vi "Convolute (Custom).vi"(6 "Kernel":dbl[][](array[numeric])=[[1.0, 2.0, 1.0], [2.0, 4.0, 2.0], [2.0, 1.0, 2.0]], 7 "Divisor":i32=1, 8 "Image Size in":T1={"Rows (X)"=256, "Colums (Y)"=256}, 9 "Paralellism":i32=2, 10 "Destination Image in":T2=refnum, 11 "Source Image Pixels (U8)":u8[][](array[numeric])) -> (2 "Destination Image Out":T2, 3 "Resulting Image Pixels (U8)":u8[][](array[numeric]))   [LabVIEW 2017, in "SoC IP Library.lvlib"]
uses:
  SoC IP Library.lvlib
  <vilib>/vision/Image Controls.llb/IMAQ Image.ctl
  Controls/Image Size.ctl
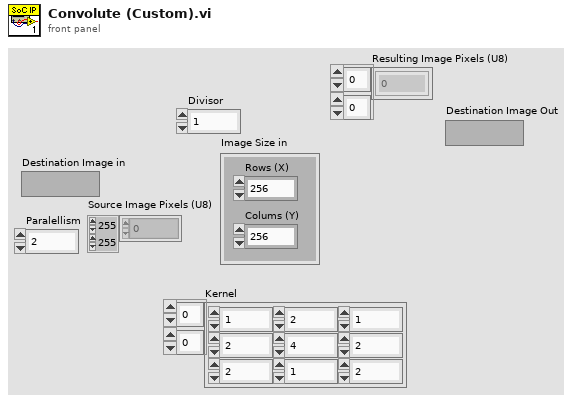
[diagram p1: front panel]
types:
  T1 = typedef "SoC IP Library.lvlib/Image Size.ctl" = cluster{"Rows (X)":u16, "Colums (Y)":u16}
  T2 = typedef "IMAQ Image.ctl" = refnum<image>
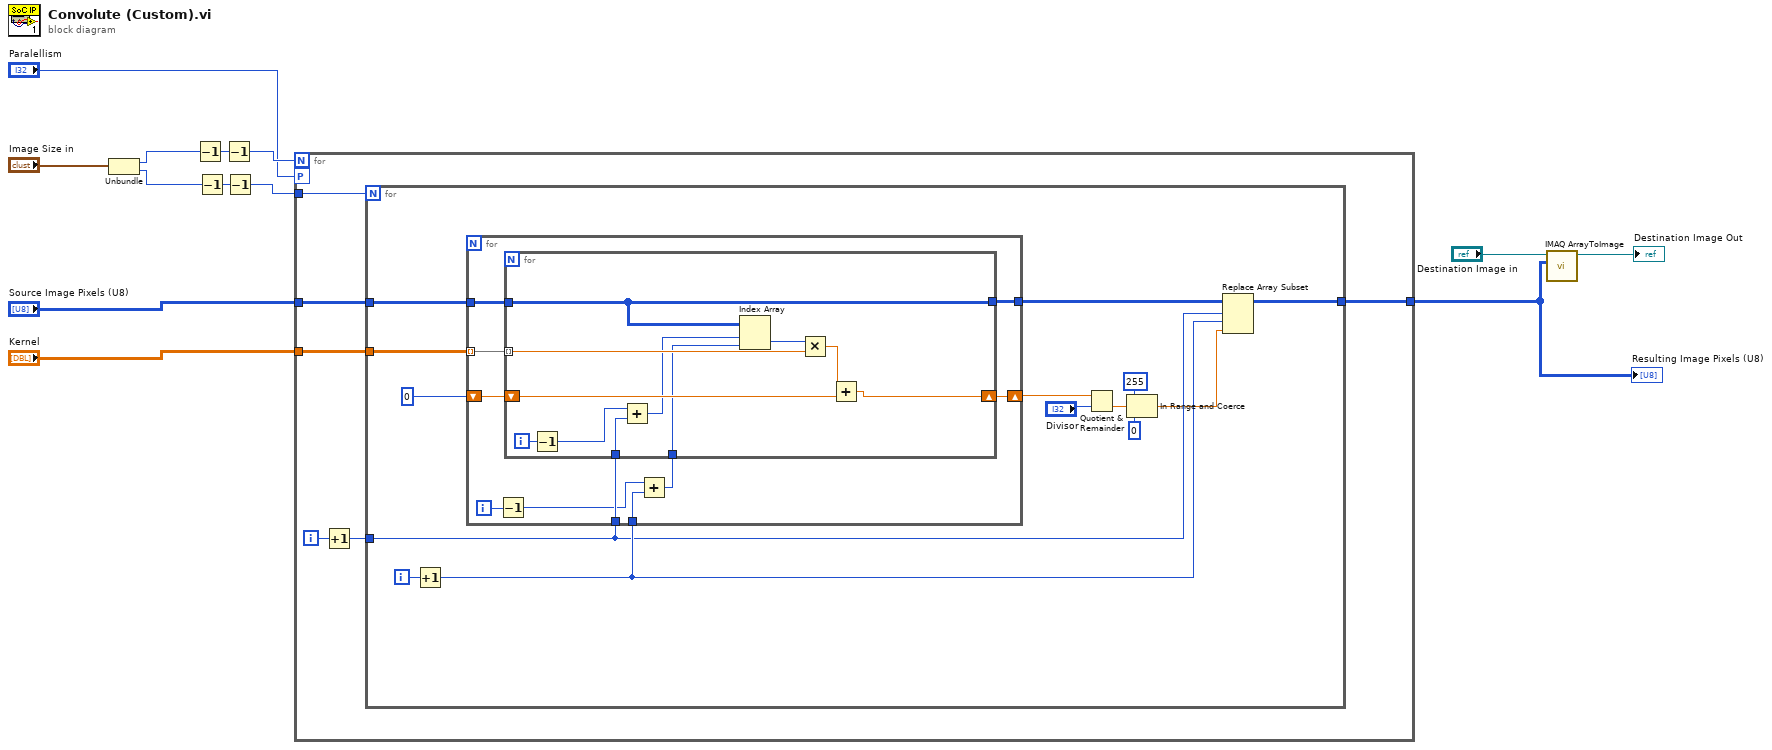
[diagram p0: block diagram]
diagram:
  n1 = Unbundle("Image Size in") -> ("Rows (X)"=w5:u16, "Colums (Y)"=w4:u16)
  n2 = Decrement(x=w5) -> (x-1=w10:u16)
  n3 = Decrement(x=w4) -> (x-1=w9:u16)
  n4 = Decrement(x=w10) -> (x-1=w12:u16)
  n5 = Decrement(x=w9) -> (x-1=w11:u16)
  n6 = for {
    N: w12 -> [_]
    tunnel: w11 -> [w19]
    tunnel: "Kernel" -> [w18]
    workers-P: "Paralellism" -> [_]
    tunnel: "Source Image Pixels (U8)" -> [w15]
    tunnel: [w14] -> w1
    i -> [w17]
    n7 = Increment(x=w17) -> (x+1=w16:i32)
    n8 = for {
      N: w19 -> [_]
      tunnel: w18 -> [w33]
      tunnel: w16 -> [w22]
      tunnel: w15 -> [w25]
      tunnel: [w20] -> w14
      i -> [w31]
      n9 = Increment(x=w31) -> (x+1=w23:i32)
      n10 = for {
        tunnel: w33 -> [w43] mode=indexing
        shift-right: [w41] -> w30
        shift-left: 0 -> [w42]
        tunnel: w23 -> [w37]
        tunnel: w22 -> [w40]
        tunnel: w25 -> [w35]
        tunnel: [w34] -> w24
        i -> [w39]
        n11 = Decrement(x=w39) -> (x-1=w38:i32)
        n12 = Add(x=w38, y=w37) -> (x+y=w36:i32)
        n13 = for {
          tunnel: w43 -> [w54] mode=indexing
          shift-right: [w51] -> w41
          shift-left: w42 -> [w52]
          tunnel: w36 -> [w46]
          tunnel: w40 -> [w49]
          tunnel: w35 -> [w44]
          tunnel: [w44] -> w34
          i -> [w50]
          n14 = Decrement(x=w50) -> (x-1=w48:i32)
          n15 = Add(x=w48, y=w49) -> (x+y=w47:i32)
          n16 = Index Array(array=w44, index (row)=w47, index (col)=w46) -> (element=w45:u8)
          n17 = Multiply(x=w45, y=w54) -> (x*y=w53:dbl)
          n18 = Add(x=w53, y=w52) -> (x+y=w51:dbl)
        }
      }
      n19 = Quotient & Remainder(x=w30, y="Divisor") -> (floor(x/y)=w29:dbl)  [unwired: 1 out]
      n20 = In Range and Coerce(upper limit=255, x=w29, lower limit=0) -> (coerced(x)=w21:dbl)  [unwired: 1 out]
      n21 = Replace Array Subset(array=w24, new element=w21, index (row)=w22, index (col)=w23) -> (w20:u8[][])
    }
  }
  "Resulting Image Pixels (U8)" <- w1
  n22 = call "IMAQ ArrayToImage"("Image Pixels (U8)"=w1, "Image"="Destination Image in") -> ("Image Out"=→"Destination Image Out":T2)  [unwired: 8 in, 1 out]
